vi "vew -- tale of three cursors.vi"() -> ()   [LabVIEW 2010]
uses:
  <vilib>/event_ctls.llb/lveventtype.ctl
  <vilib>/event_ctls.llb/eventvkey.ctl
  tale of three indices -- int -- control.ctl
  tale of three indices -- selector -- control.ctl
  command stack.vi
  tale of three indices -- check state.vi
  Q -- check range -- i -- integer.vi
  Q - not nan -- integer.vi
panel:
  out "tale of three indices -- int -- control out":T1={"left"=0, "center"=0, "right"=0, "right most"=0, "left most"=0, "window"=0, "max win factor"=2, "max win"=2, "min win"=2}
  out "at right end?":bool
  out "no success ?":bool
  out "VKey":T2
  out "Type":T3
  out "Char":i16
  in  "file path":path=path "C:/data/RUS/Experiment/ProbeTest/Probe10/YBCO_6/sweep2/May_2012/051012/299.86100K_450_3100_002_051012.bin"
  out "Plot: All":cluster{"all rows":dbl[], "all rows":dbl[]}[](graph)
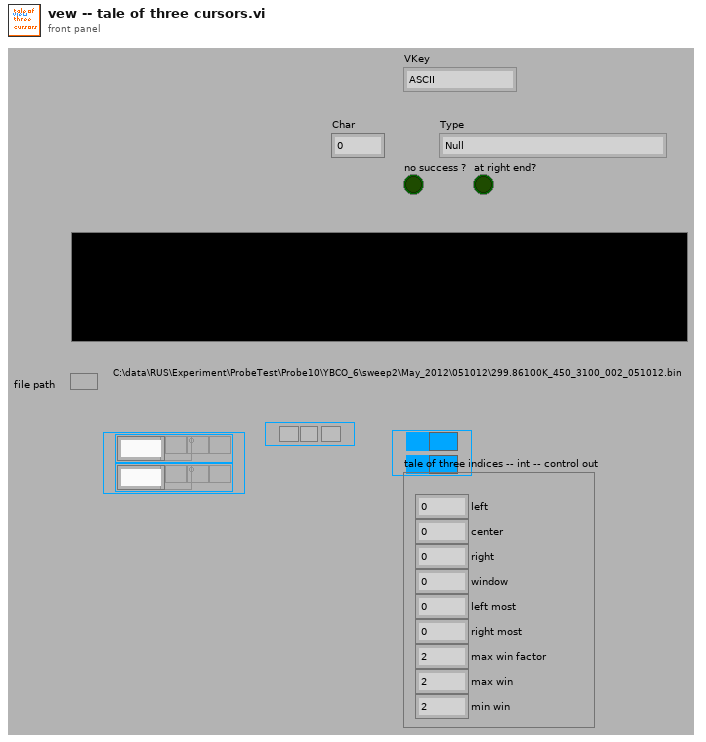
[diagram p1: front panel]
types:
  T1 = typedef "tale of three indices -- int -- control.ctl" = cluster{"left":i32, "center":i32, "right":i32, "right most":i32, "left most":i32, "window":i32, "max win factor":i32, "max win":i32, "min win":i32}
  T2 = typedef "eventvkey.ctl" = enum16{"ASCII", "Enter", "Return", "Shift", "Ctrl", "Alt", "Cmd", "Opt", "Caps", "NumLock", "Clear", "Break", "Up", "Down", "Left", "Right", "Insert", "Delete", "Home", "End", "PageUp", "PageDown", "Escape", "Help", "Pause", "ScrollLock", "F1", "F2", "F3", "F4", "F5", "F6", "F7", "F8", "F9", "F10", "F11", "F12", "F13", "F14", "F15", "F16", "F17", "F18", "F19", "F20", "F21", "F22", "F23", "F24", "Play", "VolumeUp", "VolumeDown", "Mute", "Two Byte Char"}
  T3 = typedef "lveventtype.ctl" = enum32{"Null", "Timeout", "App Instance Close", "App Instance Close?", "Autoscale Range Change", "Cell Edit", "Cell Edit?", "Cursor Grab", "Cursor Grab?", "Cursor Move", "Cursor Release", "Data Change", "Direction Change", "Display State Change", "Drag Ended", "Drag Enter", "Drag Leave", "Drag Over", "Drag Source Update", "Drag Starting", "Drag Starting?", "Drop", "Exec State Change", "Key Down", "Key Down?", "Key Repeat", "Key Repeat?", "Key Up", "Listbox Double Click", "Menu Activation?", "Menu Selection (App)", "Menu Selection? (App)", "Menu Selection (User)", "Mouse Down", "Mouse Down?", "Mouse Enter", "Mouse Leave", "Mouse Move", "Mouse Up", "NI Security User Change (App)", "Pane Size", "Panel Close", "Panel Close?", "Panel Resize", "Plot Attribute Change", "Scale Range Change", "Shortcut Menu Activation?", "Shortcut Menu Selection (App)", "Shortcut Menu Selection? (App)", "Shortcut Menu Selection (User)", "Tree Double Click", "Tree Drag", "Tree Drag?", "Tree Drop", "Tree Drop?", "Tree Item Close", "Tree Item Close?", "Tree Item Open", "Tree Item Open?", "Value Change"}
  T4 = typedef "tale of three indices -- selector -- control.ctl" = enum16{"window right", "window left", "balance", "shrink", "broaden", "do nothing", "reset", "center right", "center left", "all left", "all right", "right wing shrink", "left wing shrink", "left wing broaden", "right wing broaden", "skew left", "skew right", "check"}
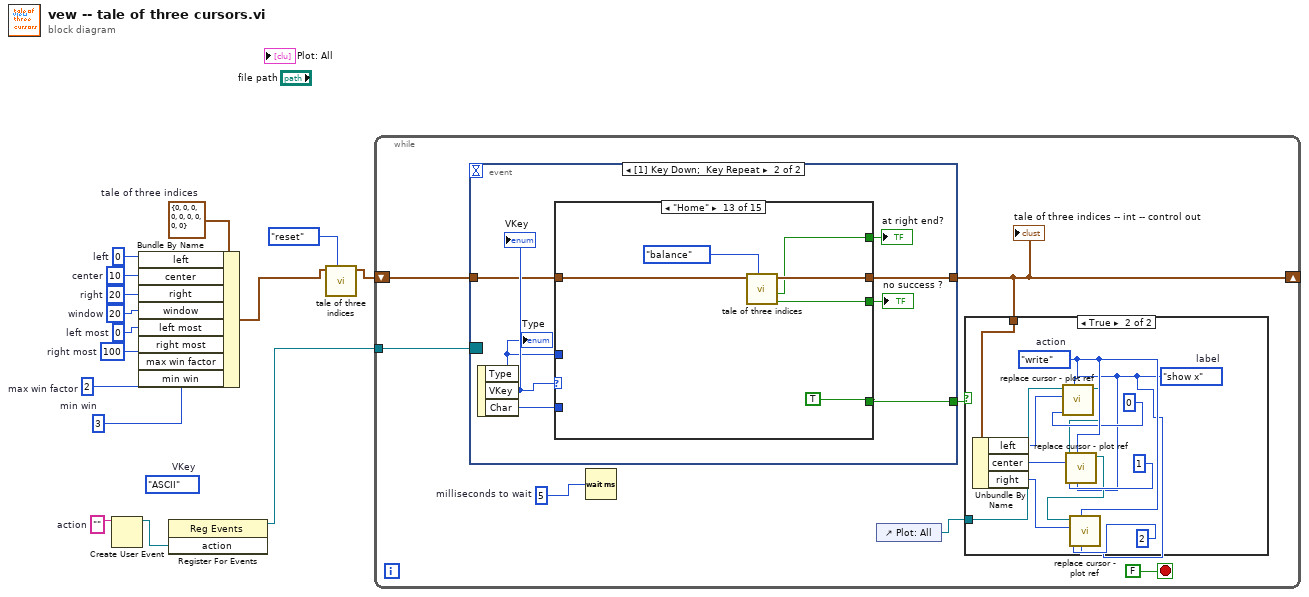
[diagram p0: block diagram]
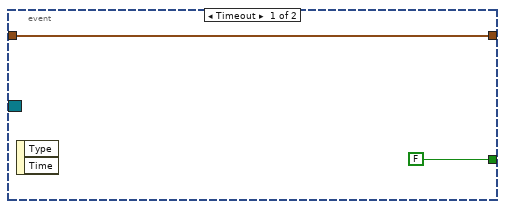
[diagram p3: hidden frame]
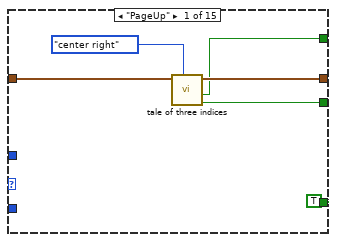
[diagram p4: hidden frame]
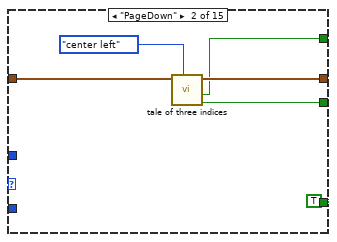
[diagram p5: hidden frame]
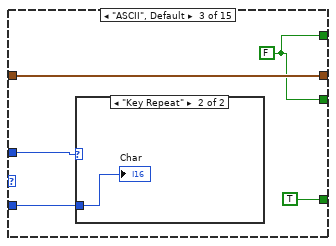
[diagram p6: hidden frame]
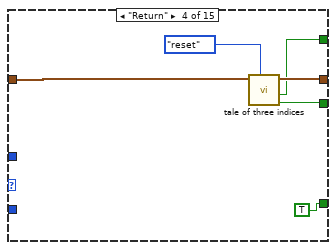
[diagram p8: hidden frame]
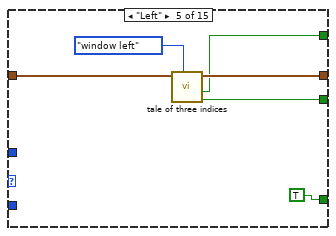
[diagram p9: hidden frame]
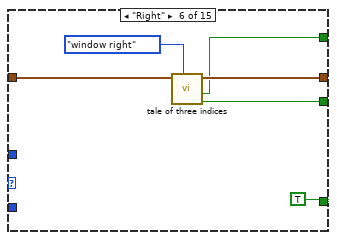
[diagram p10: hidden frame]
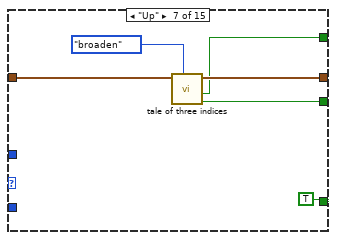
[diagram p11: hidden frame]
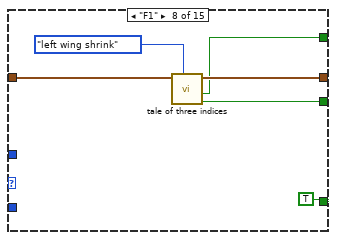
[diagram p12: hidden frame]
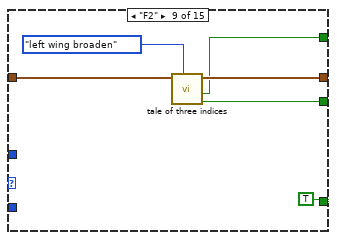
[diagram p13: hidden frame]
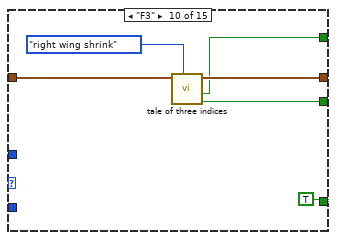
[diagram p14: hidden frame]
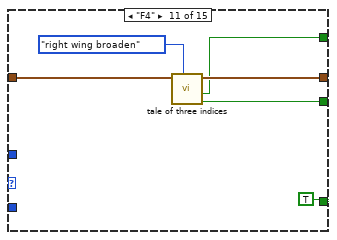
[diagram p15: hidden frame]
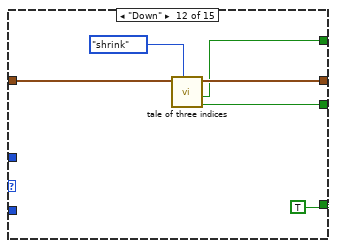
[diagram p16: hidden frame]
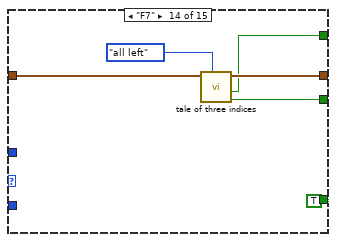
[diagram p17: hidden frame]
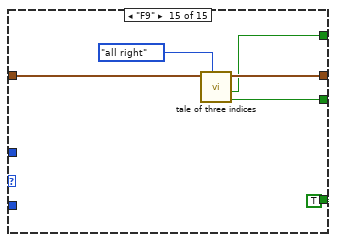
[diagram p18: hidden frame]
diagram:
  w1 = 3  # min win
  w5 = 2  # max win factor
  w12 = T1 {"left"=0, "center"=0, "right"=0, "right most"=0, "left most"=0, "window"=0, "max win factor"=0, "max win"=0, "min win"=0}  # tale of three indices
  w6 = 100  # right most
  w7 = 0  # left most
  (unwired) eventvkey."ASCII"  # VKey
  w8 = 20  # window
  w9 = 20  # right
  w11 = 0  # left
  w10 = 10  # center
  w14 = ""  # action
  n1 = Create User Event(user event datatype=w14) -> (user event=w13:refnum<user-event>)  [unwired: 1 in, 1 out]
  n2 = Bundle By Name(cluster=w12, "left"=w11, "center"=w10, "right"=w9, "window"=w8, "left most"=w7, "right most"=w6, "max win factor"=w5, "min win"=w1) -> (w3:T1)
  n3 = register-events(w13) -> (reference out=w15:refnum<event-registration>)  [unwired: 2 in, 1 out]
  n4 = call "tale of three indices.vi"("selector"=tale_of_three_indices_--_selector_--_control."reset", "tale of three indices -- int -- control"=w3) -> ("tale of three indices -- int -- control out"=w2:T1)  [unwired: 6 in, 3 out]
  n5 = while {
    tunnel: w15 -> [w22]
    shift-right: [w19] -> _
    shift-left: w2 -> [w20]
    stop <- FALSE stop-if-true
    w21 = u32 5  # milliseconds to wait
    n6 = event shown="[1] Key Down;  Key Repeat" {
      selector: w22 -> [_ _]
      dyn-events: _ -> [_ _]
      timeout: _ -> [_ _]
      tunnel: [w36 w43] -> w19
      tunnel: w20 -> [w36 w42]
      tunnel: [FALSE w40] -> w16
      event Timeout {
        n7 = event-data() -> ()  [unwired: 1 in, 2 out]
      }
      event Key Down; Key Repeat {
        n8 = event-data() -> ("Type"=w39:T3, "VKey"=w44:T2, "Char"=w41:i16)  [unwired: 1 in]
        "Type" <- w39
        "VKey" <- w44
        n9 = case shown="\"Home\"" w44 {
          tunnel: [w50 w56 w60 w66 w74 w80 w86 w92 w98 w104 w110 w116 w120 w126 w132] -> w43
          tunnel: w42 -> [w49 w55 w60 w67 w73 w79 w85 w91 w97 w103 w109 w115 w122 w128 w134]
          tunnel: w41 -> [_ _ w61 _ _ _ _ _ _ _ _ _ _ _ _]
          tunnel: [TRUE TRUE TRUE TRUE TRUE TRUE TRUE TRUE TRUE TRUE TRUE TRUE TRUE TRUE TRUE] -> w40
          tunnel: w39 -> [_ _ w58 _ _ _ _ _ _ _ _ _ _ _ _]
          tunnel: [w45 w51 w57 w63 w69 w75 w81 w87 w93 w99 w105 w111 w118 w124 w129] -> w38
          tunnel: [w46 w52 w57 w64 w70 w76 w82 w88 w94 w100 w106 w112 w117 w123 w130] -> w37
          frame "PageUp" {
            n10 = call "tale of three indices.vi"("selector"=tale_of_three_indices_--_selector_--_control."center right", "tale of three indices -- int -- control"=w49) -> ("no success ?"=w45:bool, "at right end?"=w46:bool, "tale of three indices -- int -- control out"=w50:T1)  [unwired: 6 in, 1 out]
          }
          frame "PageDown" {
            n11 = call "tale of three indices.vi"("selector"=tale_of_three_indices_--_selector_--_control."center left", "tale of three indices -- int -- control"=w55) -> ("no success ?"=w51:bool, "at right end?"=w52:bool, "tale of three indices -- int -- control out"=w56:T1)  [unwired: 6 in, 1 out]
          }
          frame "ASCII", Default {
            w57 = FALSE
            n12 = case shown="\"Key Repeat\"" w58 {
              tunnel: w61 -> [_ w62]
              frame "Null", Default {
              }
              frame "Key Repeat" {
                "Char" <- w62
              }
            }
          }
          frame "Return" {
            n13 = call "tale of three indices.vi"("selector"=tale_of_three_indices_--_selector_--_control."reset", "tale of three indices -- int -- control"=w67) -> ("no success ?"=w63:bool, "at right end?"=w64:bool, "tale of three indices -- int -- control out"=w66:T1)  [unwired: 6 in, 1 out]
          }
          frame "Left" {
            n14 = call "tale of three indices.vi"("selector"=tale_of_three_indices_--_selector_--_control."window left", "tale of three indices -- int -- control"=w73) -> ("no success ?"=w69:bool, "at right end?"=w70:bool, "tale of three indices -- int -- control out"=w74:T1)  [unwired: 6 in, 1 out]
          }
          frame "Right" {
            n15 = call "tale of three indices.vi"("selector"=tale_of_three_indices_--_selector_--_control."window right", "tale of three indices -- int -- control"=w79) -> ("no success ?"=w75:bool, "at right end?"=w76:bool, "tale of three indices -- int -- control out"=w80:T1)  [unwired: 6 in, 1 out]
          }
          frame "Up" {
            n16 = call "tale of three indices.vi"("selector"=tale_of_three_indices_--_selector_--_control."broaden", "tale of three indices -- int -- control"=w85) -> ("no success ?"=w81:bool, "at right end?"=w82:bool, "tale of three indices -- int -- control out"=w86:T1)  [unwired: 6 in, 1 out]
          }
          frame "F1" {
            n17 = call "tale of three indices.vi"("selector"=tale_of_three_indices_--_selector_--_control."left wing shrink", "tale of three indices -- int -- control"=w91) -> ("no success ?"=w87:bool, "at right end?"=w88:bool, "tale of three indices -- int -- control out"=w92:T1)  [unwired: 6 in, 1 out]
          }
          frame "F2" {
            n18 = call "tale of three indices.vi"("selector"=tale_of_three_indices_--_selector_--_control."left wing broaden", "tale of three indices -- int -- control"=w97) -> ("no success ?"=w93:bool, "at right end?"=w94:bool, "tale of three indices -- int -- control out"=w98:T1)  [unwired: 6 in, 1 out]
          }
          frame "F3" {
            n19 = call "tale of three indices.vi"("selector"=tale_of_three_indices_--_selector_--_control."right wing shrink", "tale of three indices -- int -- control"=w103) -> ("no success ?"=w99:bool, "at right end?"=w100:bool, "tale of three indices -- int -- control out"=w104:T1)  [unwired: 6 in, 1 out]
          }
          frame "F4" {
            n20 = call "tale of three indices.vi"("selector"=tale_of_three_indices_--_selector_--_control."right wing broaden", "tale of three indices -- int -- control"=w109) -> ("no success ?"=w105:bool, "at right end?"=w106:bool, "tale of three indices -- int -- control out"=w110:T1)  [unwired: 6 in, 1 out]
          }
          frame "Down" {
            n21 = call "tale of three indices.vi"("selector"=tale_of_three_indices_--_selector_--_control."shrink", "tale of three indices -- int -- control"=w115) -> ("no success ?"=w111:bool, "at right end?"=w112:bool, "tale of three indices -- int -- control out"=w116:T1)  [unwired: 6 in, 1 out]
          }
          frame "Home" {
            n22 = call "tale of three indices.vi"("selector"=tale_of_three_indices_--_selector_--_control."balance", "tale of three indices -- int -- control"=w122) -> ("no success ?"=w118:bool, "at right end?"=w117:bool, "tale of three indices -- int -- control out"=w120:T1)  [unwired: 6 in, 1 out]
          }
          frame "F7" {
            n23 = call "tale of three indices.vi"("selector"=tale_of_three_indices_--_selector_--_control."all left", "tale of three indices -- int -- control"=w128) -> ("no success ?"=w124:bool, "at right end?"=w123:bool, "tale of three indices -- int -- control out"=w126:T1)  [unwired: 6 in, 1 out]
          }
          frame "F9" {
            n24 = call "tale of three indices.vi"("selector"=tale_of_three_indices_--_selector_--_control."all right", "tale of three indices -- int -- control"=w134) -> ("no success ?"=w129:bool, "at right end?"=w130:bool, "tale of three indices -- int -- control out"=w132:T1)  [unwired: 6 in, 1 out]
          }
        }
        "no success ?" <- w38
        "at right end?" <- w37
      }
    }
    "tale of three indices -- int -- control out" <- w19
    n25 = Wait (ms)(milliseconds to wait=w21) -> ()  [unwired: 1 out]
    n26 = control-ref of="Plot: All"() -> (w18:refnum<vi>)
    n27 = case shown="True" w16 {
      tunnel: w19 -> [_ w27]
      tunnel: w18 -> [_ w29]
      frame False {
      }
      frame True {
        w23 = enum16{"hide", "show x", "show y", "show (x,y)"}."show x"  # label
        w34 = enum16{"", "read", "write"}."write"  # action
        n28 = Unbundle By Name(w27) -> ("left"=w24:i32, "center"=w26:i32, "right"=w25:i32)
        n29 = call "replace cursor - plot ref.vi"("label"=w23, "action"=w34, "cursor index"=0, "new X"=w24, "Plot ref in"=w29) -> ("Plot ref out"=w30:refnum<vi>)  [unwired: 4 in, 2 out]
        n30 = call "replace cursor - plot ref.vi"("label"=w23, "action"=w34, "cursor index"=1, "new X"=w26, "Plot ref in"=w30) -> ("Plot ref out"=w28:refnum<vi>)  [unwired: 4 in, 2 out]
        n31 = call "replace cursor - plot ref.vi"("label"=w23, "action"=w34, "cursor index"=2, "new X"=w25, "Plot ref in"=w28) -> ()  [unwired: 4 in, 3 out]
      }
    }
  }
